vi "Task_Text.vi"(8 "error in (no error)":errorcluster caption="错误输入（无错误）", 10 "事件数据":string, 11 "zsActor输入":refnum<class "zsActor.lvclass">) -> (0 "error out":errorcluster caption="错误输出", 3 "zsActor输出":refnum<class "zsActor.lvclass">)   [LabVIEW 2014, in "Wrapper.lvlib" / "zsActor.lvclass"]
uses:
  zsActor.lvclass
  zsActor.lvclass/zsActor.ctl
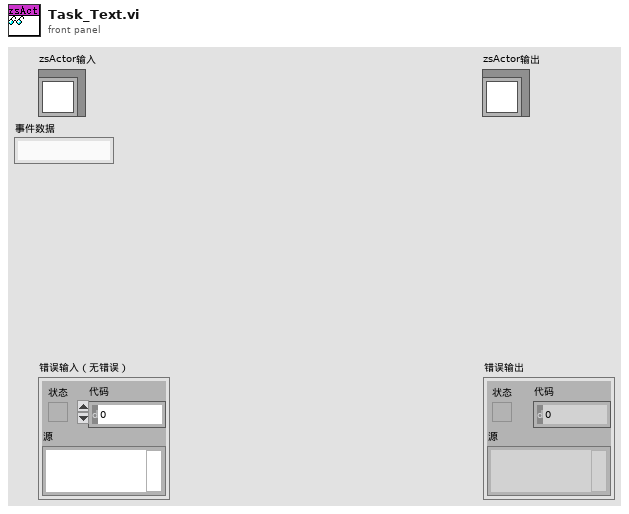
[diagram p1: front panel]
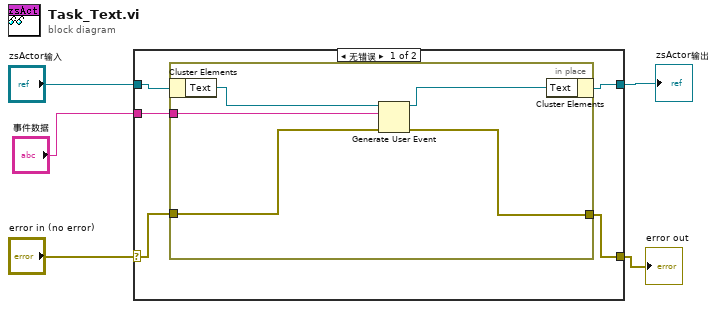
[diagram p0: block diagram]
diagram:
  n1 = case shown="无错误" "error in (no error)" {
    selector: "error in (no error)" -> [w9 w16]
    tunnel: [w8 w16] -> w4
    tunnel: [w7 w17] -> w2
    tunnel: "zsActor输入" -> [w10 w17]
    tunnel: "事件数据" -> [w6 _]
    frame No Error {
      n2 = in-place {
        in-place-border: w9 -> [w13]
        in-place-border: [w12] -> w8
        in-place-border: w6 -> [w11]
        n3 = in-place-cluster #1(w10) -> ("Text"=w15:refnum<user-event>)
        n4 = Generate User Event(user event=w15, event data cluster=w11, error in=w13) -> (user event out=w14:refnum<user-event>, error out=w12:errorcluster)  [unwired: 1 in]
        n5 = in-place-cluster #1("Text"=w14) -> (w7:refnum<class "zsActor.lvclass">)
      }
    }
    frame Error {
    }
  }
  "error out" <- w4
  "zsActor输出" <- w2
